vi "RT Driver VI.vi"(7 "Operation":T1, 11 "Device Reference in":T2 format="%.0x") -> (0 "Error Code":i32)   [LabVIEW 2026, in "WebPage Addon Engine.lvlib"]
uses:
  WebPage Addon Engine.lvlib
  <vilib>/NI VeriStand/Custom Device API/Custom Device Item Ref.ctl
  <vilib>/NI VeriStand/Custom Device API/Hardware Interface Driver VI Operation.ctl
  Shared/Compiled.Settings.ctl
  <vilib>/NI/NIVS Inline Async API/_VS Inline Async API/VS Inline Async API/VS Inline Async API.lvclass
  <vilib>/NI/NIVS Inline Async API/_VS Inline Async API/VS Inline Async API/VS Inline Async API.lvclass/VS Inline Async API.ctl
  <vilib>/NI/NIVS Inline Async API/_Data Access Engine/Data Access Engine/Data Access Engine.lvclass/Data Access Engine.ctl
  <vilib>/NI/NIVS Inline Async API/_Data Access Engine/Access Type Classes/Write/Write.lvclass/Write.ctl
  <vilib>/NI/NIVS Inline Async API/_Data Access Engine/Access Type Classes/ReadWrite/ReadWrite.lvclass/ReadWrite.ctl
  <vilib>/NI/NIVS Inline Async API/_Data Access Engine/Access Type Classes/Read/Read.lvclass/Read.ctl
  <vilib>/NI/NIVS Inline Async API/_Data Access Engine/Data Access Engine/Methods/Data.Engine.Read Data from HW.vi
  <vilib>/NI/NIVS Inline Async API/_VS Inline Async API/Error Handling Process/SubVIs/Error.GetError.vi
  <vilib>/NI/NIVS Inline Async API/_Data Access Engine/Data Access Engine/Methods/Data.Engine.Write Data to HW.vi
  <vilib>/NI/NIVS Inline Async API/_Data Access Engine/Access Type Classes/ReadWrite/ReadWrite.EngineData.vi
  <vilib>/NI/NIVS Inline Async API/_Data Access Engine/Access Type Classes/Write/Write.EngineData.vi
  <vilib>/NI/NIVS Inline Async API/_Data Access Engine/Access Type Classes/Read/Read.EngineData.vi
  <vilib>/NI VeriStand/Custom Device API/NI VeriStand - Get Channel Value by Data Reference.vi
  <vilib>/NI VeriStand/Custom Device API/NI VeriStand - Set Channel Value by Data Reference.vi
  <vilib>/NI VeriStand/Custom Device API/NI VeriStand - Set Channel Values by Block Data Reference.vi
  <vilib>/NI VeriStand/Custom Device API/NI VeriStand - Get Channel Values by Block Data Reference.vi
  WebPage-Custom-Device.Async.vi
  Shared/Constants.vi
  <vilib>/NI VeriStand/Custom Device API/Get Item Property (Variant).vi
  <vilib>/NI VeriStand/Custom Device API/Global Data Refs.vi
  <vilib>/NI VeriStand/Custom Device API/Custom Device API.lvlib
  <vilib>/NI VeriStand/Custom Device Tools/Custom Device Utility Library/Custom Device Utility Library.lvlib
  Shared/WebPage Addon Shared.lvlib
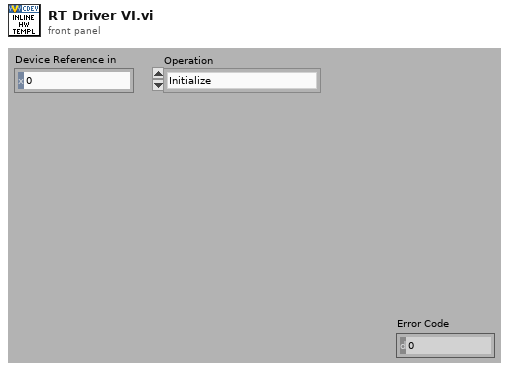
[diagram p1: front panel]
types:
  T1 = typedef "Custom Device API.lvlib/Hardware Interface Driver VI Operation.ctl" = enum16{"Initialize", "Start", "Read Data from HW", "Write Data to HW", "Close"}
  T2 = typedef "Custom Device API.lvlib/Custom Device Item Ref.ctl" = u64
  T3 = typedef "WebPage Addon Shared.lvlib/Compiled.Settings.ctl" = cluster{"Name":string, "Decimation":u32, "Channel Names":string[]}
  T4 = cluster{"Async":refnum<class "VS Inline Async API.lvclass">, "Settings":T3, "Iteration Count":i32}
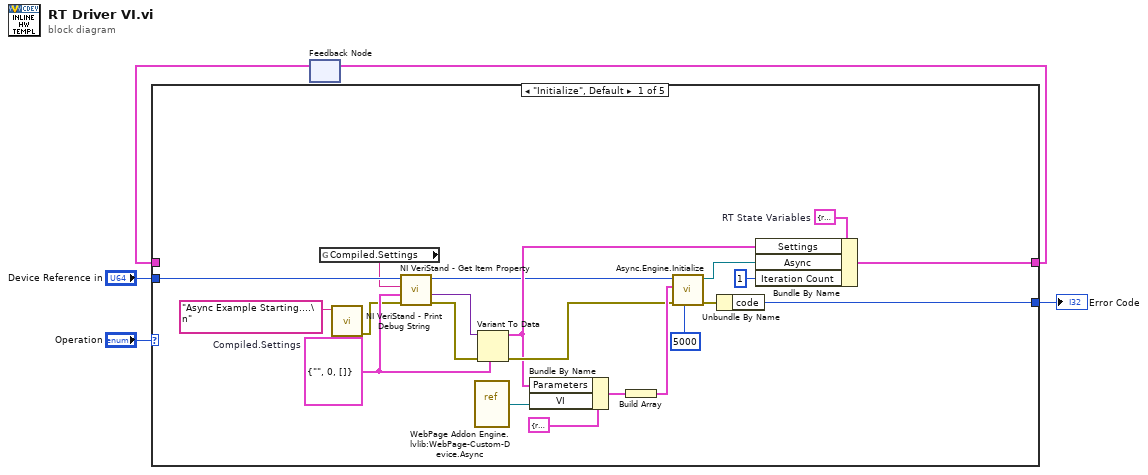
[diagram p0: block diagram]
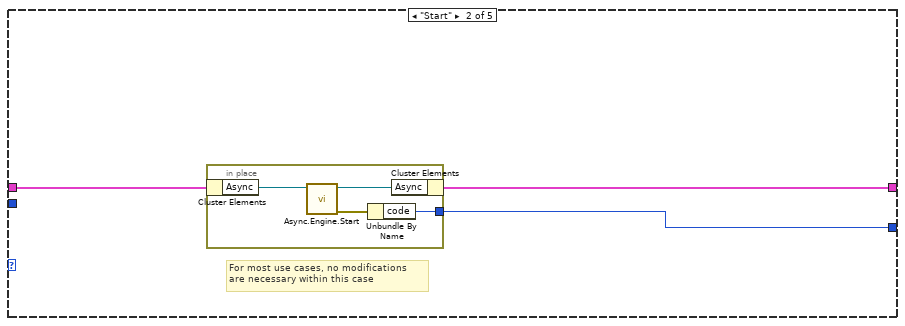
[diagram p2: hidden frame]
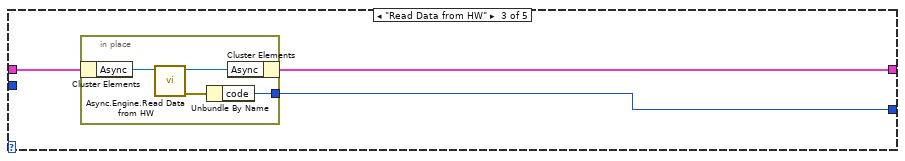
[diagram p3: hidden frame]
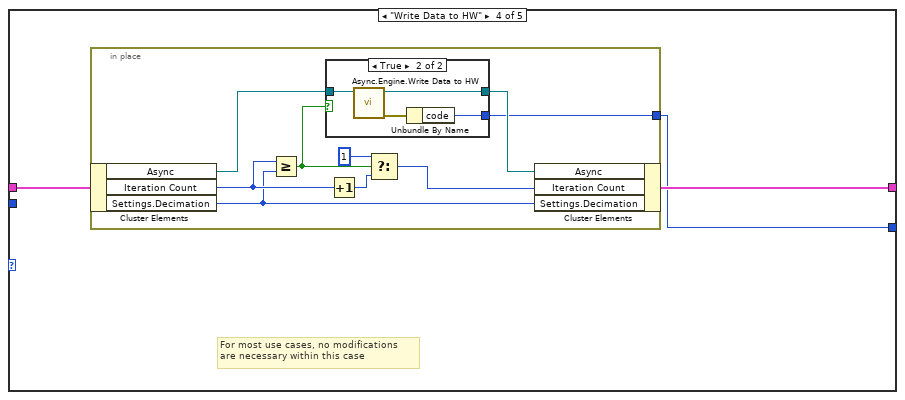
[diagram p4: hidden frame]
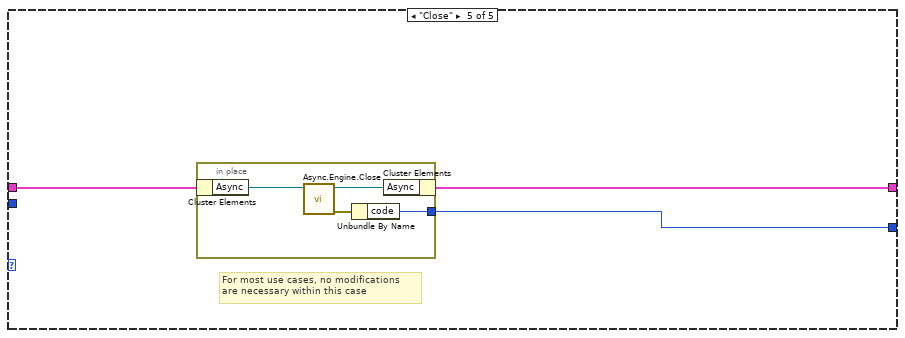
[diagram p6: hidden frame]
diagram:
  n1 = feedback #1() -> (w3:T4)  [unwired: 1 out]
  n2 = case shown="\"Initialize\", Default" "Operation" {
    tunnel: [w24 w28 w34 w42 w59] -> w4
    tunnel: w3 -> [_ w29 w35 w43 w60]
    tunnel: "Device Reference in" -> [w21 _ _ _ _]
    tunnel: [w26 w27 w36 w41 w58] -> w1
    frame "Initialize", Default {
      w16 = T4 {"Async"=refnum, "Settings"={"Name"="", "Decimation"=0, "Channel Names"=[]}, "Iteration Count"=0}  # RT State Variables
      w17 = T3 {"Name"="", "Decimation"=0, "Channel Names"=[]}  # Compiled.Settings
      n3 = global read "Constants.vi" "Compiled.Settings"() -> (w18:string)
      n4 = call <vilib>:"NI VeriStand - Print Debug String.vi"("Message"="Async Example Starting....\n") -> ("error out"=w13:errorcluster)  [unwired: 10 in]
      n5 = call-poly <vilib>:"NI VeriStand - Get Item Property.vi"("error in (no error)"=w13, "Default Value"=w17, "Property Name"=w18, "Item Ref in"=w21) -> ("error out"=w20:errorcluster, "Value"=w19:variant, "Item Ref out"=w8:T2)  [unwired: 4 in, 1 out]
      n6 = vi-ref "WebPage Addon Engine.lvlib:WebPage-Custom-Device.Async.vi"() -> (w11:refnum<vi>)
      n7 = Variant To Data(error in=w20, type=w17, Variant=w19) -> (data=w10:T3, error out=w14:errorcluster)
      n8 = Bundle By Name(cluster=cluster{"VI":refnum<vi>, "Parameters":variant} {"VI"=refnum, "Parameters"=variant} ("Process"), "Parameters"=w10, "VI"=w11) -> (w22:cluster{"VI":refnum<vi>, "Parameters":variant})
      n9 = Build Array(w22) -> (w15:cluster{"VI":refnum<vi>, "Parameters":variant}[])
      n10 = call <vilib>:"Async.Engine.Initialize.vi"("Timeout (ms) (5000)"=u16 5000, "error in (no error)"=w14, "Processes"=w15, "Custom Device Ref"=w8) -> ("error out"=w9:errorcluster, "Async"=w25:refnum<class "VS Inline Async API.lvclass">)  [unwired: 6 in]
      n11 = Unbundle By Name(w9) -> ("code"=w26:i32)
      n12 = Bundle By Name(cluster=w16, "Settings"=w10, "Async"=w25, "Iteration Count"=1) -> (w24:T4)
    }
    frame "Start" {
      # "For most use cases, no modifications \nare necessary within this case"
      n13 = in-place {
        in-place-border: [w30] -> w27
        n14 = in-place-cluster #2(w29) -> ("Async"=w33:refnum<class "VS Inline Async API.lvclass">)
        n15 = call <vilib>:"Async.Engine.Start.vi"("VS Inline Async API in"=w33) -> ("error out"=w31:errorcluster, "VS Inline Async API out"=w32:refnum<class "VS Inline Async API.lvclass">)  [unwired: 9 in]
        n16 = Unbundle By Name(w31) -> ("code"=w30:i32)
        n17 = in-place-cluster #2("Async"=w32) -> (w28:T4)
      }
    }
    frame "Read Data from HW" {
      n18 = in-place {
        in-place-border: [w40] -> w36
        n19 = in-place-cluster #3(w35) -> ("Async"=w38:refnum<class "VS Inline Async API.lvclass">)
        n20 = call <vilib>:"Async.Engine.Read Data from HW.vi"("Async in"=w38) -> ("error out"=w39:errorcluster, "Async out"=w37:refnum<class "VS Inline Async API.lvclass">)  [unwired: 9 in]
        n21 = Unbundle By Name(w39) -> ("code"=w40:i32)
        n22 = in-place-cluster #3("Async"=w37) -> (w34:T4)
      }
    }
    frame "Write Data to HW" {
      # "For most use cases, no modifications \nare necessary within this case"
      n23 = in-place {
        in-place-border: [w50] -> w41
        n24 = in-place-cluster #4(w43) -> ("Async"=w52:refnum<class "VS Inline Async API.lvclass">, "Iteration Count"=w47:i32, "Settings.Decimation"=w44:u32)
        n25 = Greater Or Equal?(x=w47, y=w44) -> (x >= y?=w49:bool)
        n26 = case shown="True" w49 {
          tunnel: w52 -> [w53 w56]
          tunnel: [w53 w54] -> w51
          tunnel: [_ w57] -> w50
          frame False {
          }
          frame True {
            n27 = call <vilib>:"Async.Engine.Write Data to HW.vi"("VS Inline Async API in"=w56) -> ("error out"=w55:errorcluster, "VS Inline Async API out"=w54:refnum<class "VS Inline Async API.lvclass">)  [unwired: 9 in]
            n28 = Unbundle By Name(w55) -> ("code"=w57:i32)
          }
        }
        n29 = Increment(x=w47) -> (x+1=w46:i32)
        n30 = Select(t=1 ("Iteration Count"), s=w49, f=w46) -> (s? t:f=w45:i32)
        n31 = in-place-cluster #4("Async"=w51, "Iteration Count"=w45, "Settings.Decimation"=w44) -> (w42:T4)
      }
    }
    frame "Close" {
      # "For most use cases, no modifications \nare necessary within this case"
      n32 = in-place {
        in-place-border: [w62] -> w58
        n33 = in-place-cluster #5(w60) -> ("Async"=w64:refnum<class "VS Inline Async API.lvclass">)
        n34 = call <vilib>:"Async.Engine.Close.vi"("Async in"=w64) -> ("error out"=w61:errorcluster, "Async out"=w63:refnum<class "VS Inline Async API.lvclass">)  [unwired: 9 in]
        n35 = Unbundle By Name(w61) -> ("code"=w62:i32)
        n36 = in-place-cluster #5("Async"=w63) -> (w59:T4)
      }
    }
  }
  "Error Code" <- w1
  n37 = feedback-in #1(w4) -> ()
